vi "Read Prep.vi"(8 "error in (no error)":errorcluster, 11 "Photon Counter SR400 in":refnum<class "Photon Counter.lvclass">) -> (0 "error out":errorcluster, 3 "Photon Counter SR400 out":refnum<class "Photon Counter.lvclass">)   [LabVIEW 2017, in "Photon Counter.lvclass"]
doc: "This is in case the readable object needs to change some settings before the time delay occurs. One example: if the photon counter needs to change the gates, e.g. to track the current pulse settings."
uses:
  Photon Counter.lvclass
  Utility Classes/Readable/Readable.lvclass
  SR400/SR400.lvlib
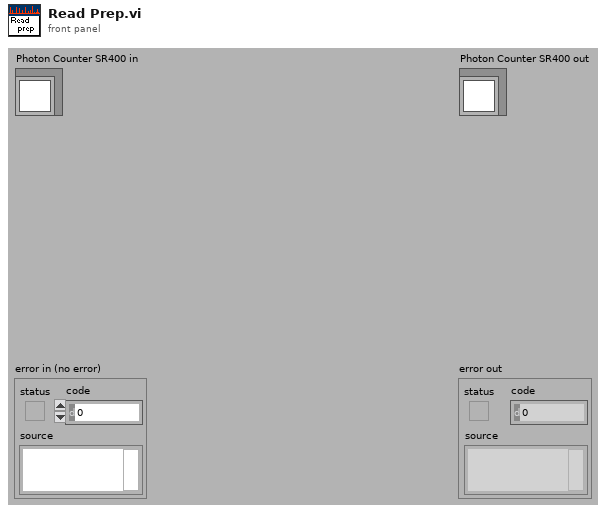
[diagram p1: front panel]
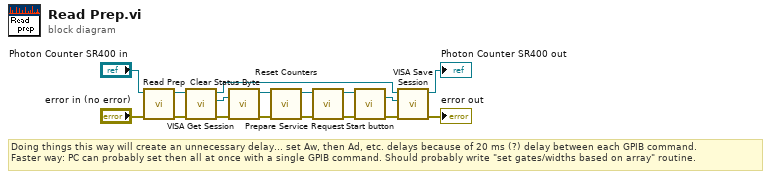
[diagram p0: block diagram]
diagram:
  # "Doing things this way will create an unnecessary delay... set Aw, then Ad, etc. delays because of 20 ms (?) delay between each GPIB command.\nFaster way: PC can probably set then all at once with a single GPIB command. Should probably write \"set gates/widths based on array\" routine."
  n1 = call-parent "Read Prep.vi"("error in (no error)"="error in (no error)", "Readable in"="Photon Counter SR400 in") -> ("error out"=w9:errorcluster, "Readable out"=w10:refnum<class "Photon Counter.lvclass">)  [unwired: 8 out]
  n2 = call-dynamic "VISA Get Session.vi"("error in (no error)"=w9, "Instrument.lvclass in"=w10) -> ("error out"=w3:errorcluster, "VISA Resource Name"=w4:refnum<visa-resource-name>, "Instrument.lvclass out"=w5:refnum<class "Photon Counter.lvclass">)  [unwired: 7 out]
  n3 = call "Clear Status Byte.vi"("error in (no error)"=w3, "VISA resource name"=w4) -> ("error out"=w13:errorcluster, "VISA resource name out"=w16:refnum<visa-resource-name>)  [unwired: 8 out]
  n4 = call "Reset Counters.vi"("error in (no error)"=w13, "VISA resource name"=w16) -> ("error out"=w12:errorcluster, "VISA resource name out"=w15:refnum<visa-resource-name>)  [unwired: 8 out]
  n5 = call "Prepare Service Request.vi"("error in (no error)"=w12, "VISA resource name"=w15) -> ("error out"=w11:errorcluster, "VISA resource name out"=w14:refnum<visa-resource-name>)  [unwired: 1 in, 7 out]
  n6 = call "Start button.vi"("error in (no error)"=w11, "VISA resource name"=w14) -> ("error out"=w6:errorcluster, "VISA resource name out"=w7:refnum<visa-resource-name>)  [unwired: 8 out]
  n7 = call-dynamic "VISA Save Session.vi"("error in (no error)"=w6, "VISA Resource Name"=w7, "Instrument.lvclass in"=w5) -> ("error out"=→"error out":errorcluster, "Instrument.lvclass out"=→"Photon Counter SR400 out":refnum<class "Photon Counter.lvclass">)  [unwired: 7 out]
